vi "AddNumRow (SubVI).vi"(10 "element":i32, 11 "Table in":refnum<vi>) -> ()   [LabVIEW 2017]
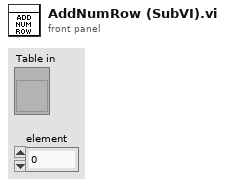
[diagram p1: front panel]
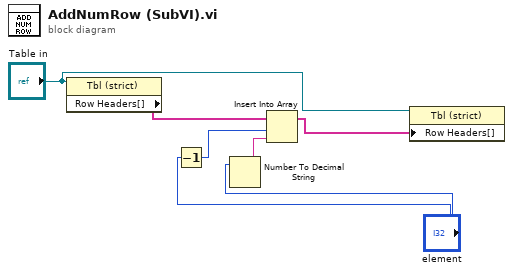
[diagram p0: block diagram]
diagram:
  n1 = property on="Property Node" class="Tbl (strict)"(reference="Table in") -> ("Row Headers[]"=w5:string[])  [unwired: 1 in, 2 out]
  n2 = Decrement(x="element") -> (x-1=w2:i32)
  n3 = Number To Decimal String(number="element") -> (decimal integer string=w4:string)  [unwired: 1 in]
  n4 = Insert Into Array(array=w5, index=w2, new element=w4) -> (w3:string[])
  n5 = property on="Property Node" class="Tbl (strict)"(reference="Table in", "Row Headers[]"=w3) -> ()  [unwired: 1 in, 2 out]
